vi "TEST NEW VIs.vi"() -> ()   [LabVIEW 2020]
uses:
  library/LVData/variant.lvclass
  library/openg_variant.lvlib
  library/variant.lvlib
  library/LVData/Type Descriptor/TD.lvclass
panel:
  out "error out 2":errorcluster
  out "Data out 4":variant
  out "Element Names":string[](array[string])
  out "name 2":string
  out "name":string
  out "enum name":string
  out "enum strings 2":string[](array[string])
  out "enum strings":string[](array[string])
  out "Data out 3":variant
  out "error out":errorcluster
  out "Data out":variant
  out "Renamed Data":variant
  out "Data out 2":variant
  out "set data name?":bool
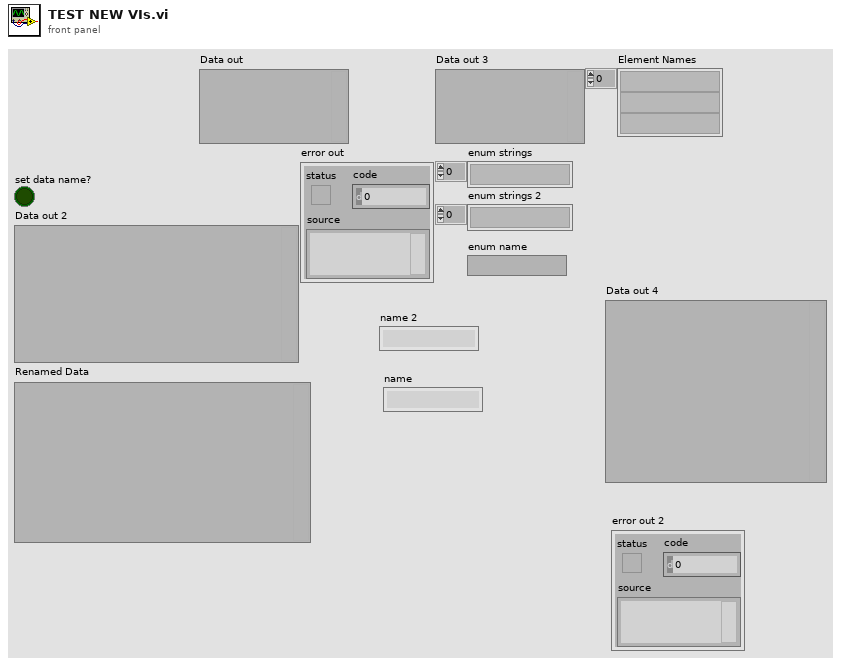
[diagram p1: front panel]
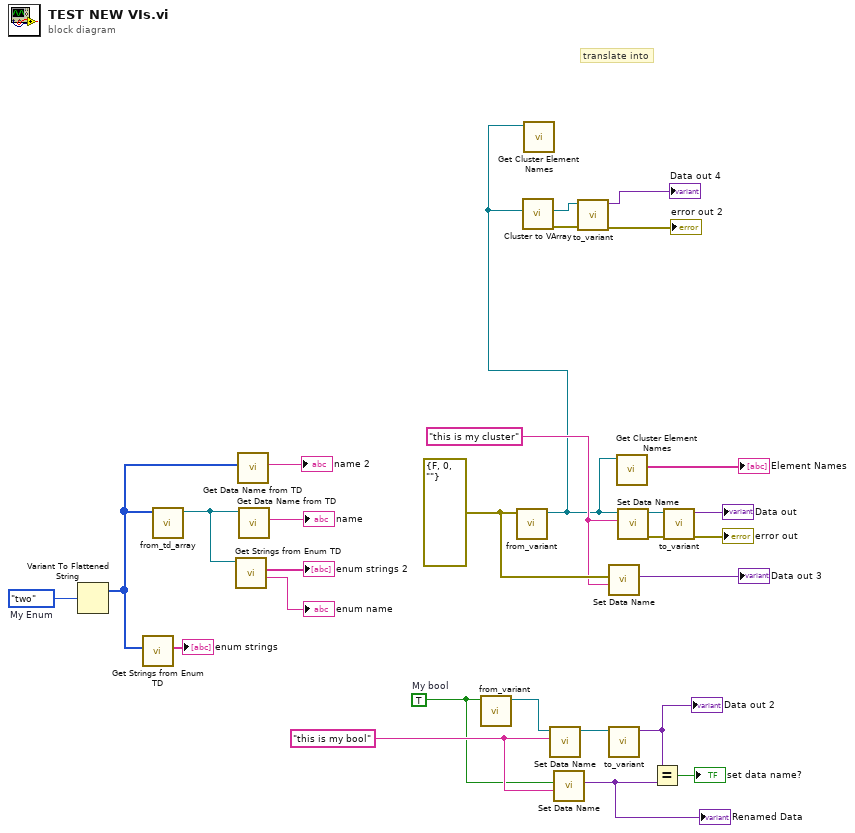
[diagram p0: block diagram]
diagram:
  w14 = enum16{"one", "two", "three"}."two"  # My Enum
  w16 = "this is my cluster" ("Data Name")
  w17 = errorcluster {"status"=FALSE, "code"=0, "source"=""} ("error constant")
  w27 = "this is my bool" ("Data Name")
  w22 = TRUE  # My bool
  # "translate into"
  n1 = Variant To Flattened String(Variant=w14) -> (1:w9:i16[])  [unwired: 1 out]
  n2 = call "Get Strings from Enum TD.vi"("Type Descriptor"=w9) -> ("enum strings"=→"enum strings":string[])  [unwired: 8 in, 2 out]
  n3 = call "from_td_array.vi"("type descriptor array"=w9) -> ("TypeDescriptor out"=w7:refnum<class "TD.lvclass">)  [unwired: 9 in, 1 out]
  n4 = call "Get Strings from Enum TD.vi"("Type Descriptor"=w7) -> ("enum name"=→"enum name":string, "enum strings"=→"enum strings 2":string[])  [unwired: 7 in, 2 out]
  n5 = call "Get Data Name from TD.vi"("Type Descriptor"=w9) -> ("name"=→"name 2":string)  [unwired: 9 in, 1 out]
  n6 = call "Get Data Name from TD.vi"("TypeDescriptor"=w7) -> ("name"=→"name":string)  [unwired: 8 in, 2 out]
  n7 = call "from_variant.vi"("Data"=w22) -> ("LVData out"=w28:refnum<class "variant.lvclass">)  [unwired: 9 in, 1 out]
  n8 = call "from_variant.vi"("Data"=w17) -> ("LVData out"=w5:refnum<class "variant.lvclass">)  [unwired: 9 in, 1 out]
  n9 = call "Cluster to VArray.vi"("Cluster"=w5) -> ("error out"=w2:errorcluster, "VArray"=w4:refnum<class "variant.lvclass">)  [unwired: 9 in]
  n10 = call "Get Cluster Element Names.vi"("LVData"=w5) -> ()  [unwired: 8 in, 3 out]
  n11 = call "Set Data Name.vi"("Data Name"=w27, "LVData in"=w28) -> ("LVData out"=w26:refnum<class "variant.lvclass">)  [unwired: 8 in, 1 out]
  n12 = call "Set Data Name.vi"("Data Name"=w27, "Data"=w22) -> ("Renamed Data"=w25:variant)  [unwired: 8 in, 1 out]
  "Renamed Data" <- w25
  n13 = call "to_variant.vi"("error in (no error)"=w2, "LVData in"=w4) -> ("error out"=→"error out 2":errorcluster, "Data out"=→"Data out 4":variant)  [unwired: 8 in]
  n14 = call "Set Data Name.vi"("Data Name"=w16, "Data"=w17) -> ("Renamed Data"=→"Data out 3":variant)  [unwired: 8 in, 1 out]
  n15 = call "to_variant.vi"("LVData in"=w26) -> ("Data out"=w24:variant)  [unwired: 9 in, 1 out]
  "Data out 2" <- w24
  n16 = call "Get Cluster Element Names.vi"("LVData"=w5) -> ("Element Names"=→"Element Names":string[])  [unwired: 8 in, 2 out]
  n17 = call "Set Data Name.vi"("Data Name"=w16, "LVData in"=w5) -> ("error out"=w18:errorcluster, "LVData out"=w21:refnum<class "variant.lvclass">)  [unwired: 8 in]
  n18 = Equal?(x=w24, y=w25) -> (x = y?=→"set data name?":bool)
  n19 = call "to_variant.vi"("error in (no error)"=w18, "LVData in"=w21) -> ("error out"=→"error out":errorcluster, "Data out"=→"Data out":variant)  [unwired: 8 in]
